vi "Read Average.vi"(11 "Power Meter in":refnum<class "Power Meter.lvclass">) -> (2 "Average":cluster{"Average":i32, "Average State":bool}, 3 "Power Meter out":refnum<class "Power Meter.lvclass">)   [LabVIEW 2020, in "Power Meter.lvclass"]
uses:
  Power Meter.lvclass
  Power Meter.lvclass/Power Meter.ctl
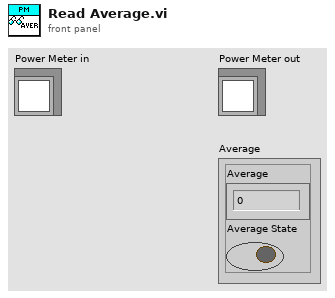
[diagram p1: front panel]
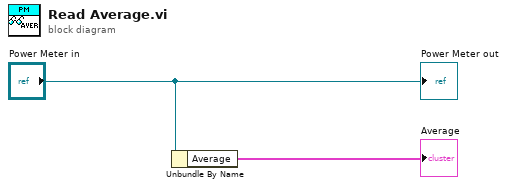
[diagram p0: block diagram]
diagram:
  n1 = Unbundle By Name("Power Meter in") -> ("Average"=→"Average":cluster{"Average":i32, "Average State":bool})
  "Power Meter out" <- "Power Meter in"
